vi "SVPO Average Power Spectrum (Real).vi"   [LabVIEW 2017]
doc: "Computes linear RMS-averaged power spectrum of instantaneous input power spectrum. Use this VI when you require more flexibility to compute multiple/different averages while reusing the same implementation of the device under test [DUT]."
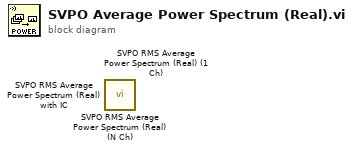
[diagram p0: block diagram]
diagram:
  n1 = call <vilib>:"SVPO RMS Average Power Spectrum (Real) (N Ch).vi"() -> ()  [unwired: 17 in, 3 out]
  n2 = call <vilib>:"SVPO RMS Average Power Spectrum (Real) (1 Ch).vi"() -> ()  [unwired: 17 in, 3 out]
  n3 = call <vilib>:"SVPO RMS Average Power Spectrum (Real) with IC.vi"() -> ()  [unwired: 17 in, 3 out]
